vi "MSTSoftwareBinDamage.vi"() -> ()   [LabVIEW 2012]
uses:
  <vilib>/addons/database/Auxilliary.llb/DB Tools Cursor Type.ctl
  <vilib>/addons/database/Connection.llb/DB Tools Open Connec (Path).vi
  <vilib>/addons/database/Connection.llb/Conn Execute.vi
  <vilib>/addons/database/Recordset.llb/Rec Fetch Recordset Data (R).vi
  <vilib>/addons/database/Recordset.llb/Rec Destroy - Connection.vi
  <vilib>/addons/database/Recordset.llb/Rec Fetch Integer Data (R).vi
  <vilib>/addons/database/_DB Variant To Data/Database Variant To Data.xnode
  <vilib>/addons/database/NI_Database_API.lvlib
panel:
  out "concatenated string 3":string
  out "concatenated string 2":string
  out "concatenated string":string
  out "error out 2":errorcluster
  out "recordset data":variant[][](array[variant])
  out "data":string
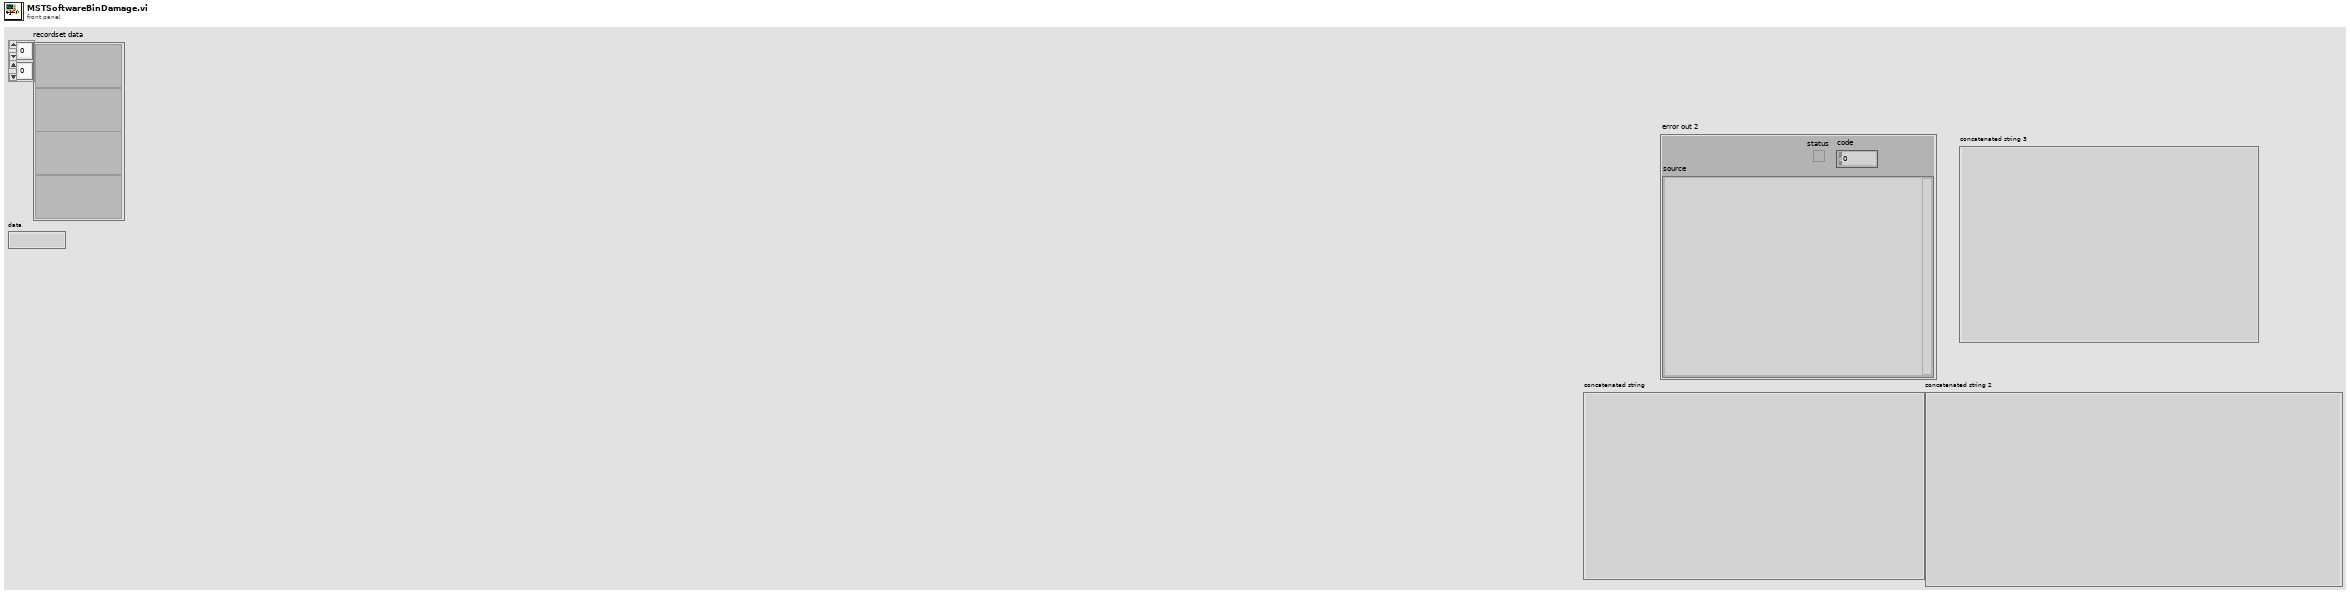
[diagram p1: front panel]
types:
  T1 = typedef "NI_Database_API.lvlib/DB Tools Cursor Type.ctl" = enum16{"forward-only", "keyset", "dynamic", "static"}
  T2 = typedef "NI_Database_API.lvlib/Conn ObjectReference.ctl" = refnum<k1>
  T3 = typedef "NI_Database_API.lvlib/Rec ObjectReference.ctl" = refnum<k1>
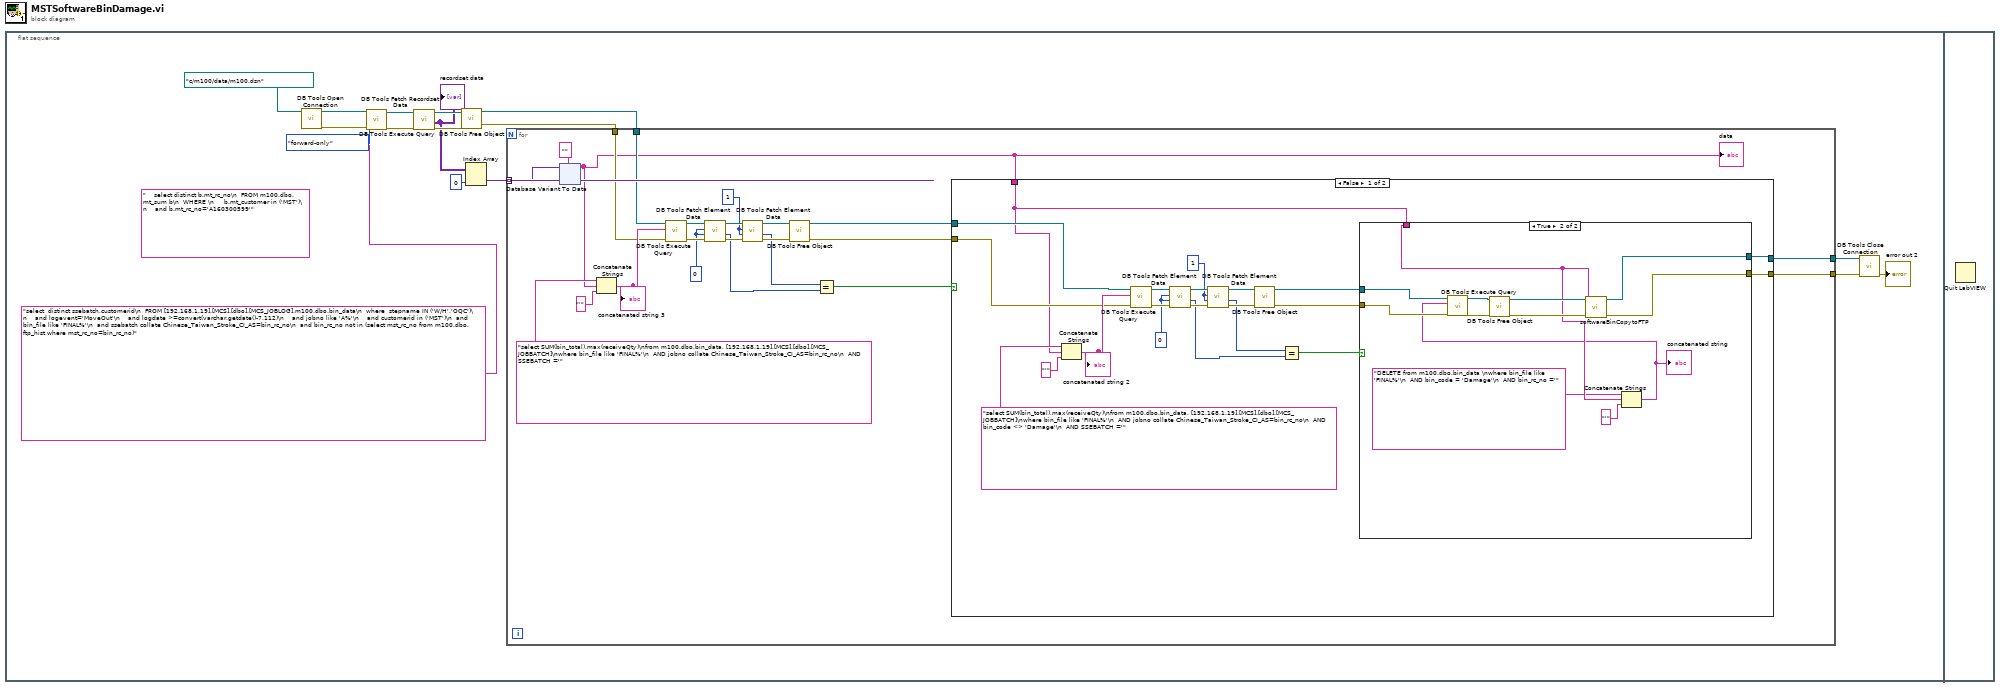
[diagram p0: block diagram]
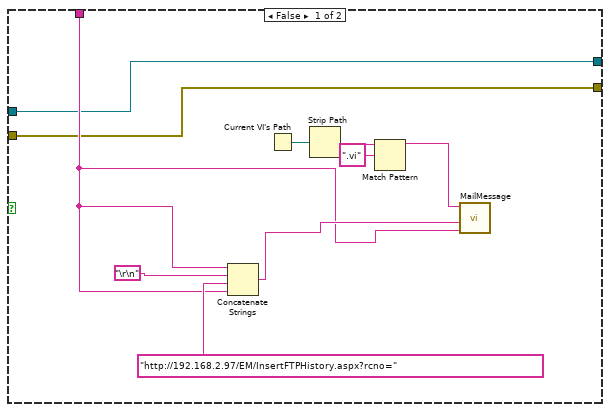
[diagram p2: hidden frame]
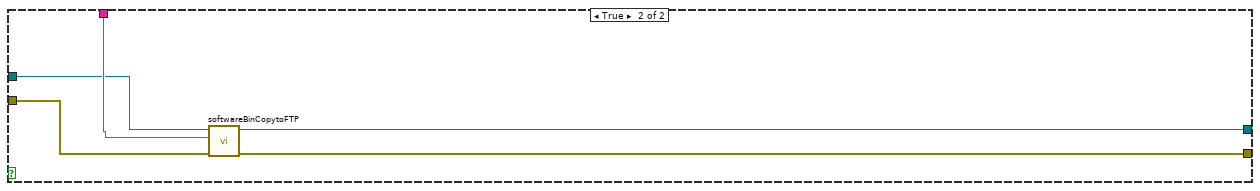
[diagram p3: hidden frame]
diagram:
  n1 = flat-sequence {
    frame #0 {
      (unwired) "    select distinct b.mt_rc_no\n  FROM m100.dbo.mt_sum b\n  WHERE \n     b.mt_customer in ('MST')\n    and b.mt_rc_no='A160300599'" ("SQL query")
      n2 = call-poly <vilib>:"DB Tools Open Connection.vi"("connection information"=path "c:/m100/data/m100.dsn") -> ("error out"=w14:errorcluster, "connection reference"=w17:T2)  [unwired: 7 in]
      n3 = call-poly <vilib>:"DB Tools Execute Query.vi"("error in (no error)"=w14, "cursor type"=DB_Tools_Cursor_Type."forward-only", "SQL query"="select  distinct ssebatch,customerid\n  FROM [192.168.1.19].[MCS].[dbo].[MCS_JOBLOG],m100.dbo.bin_data\n  where  stepname IN ('W/H','OQC')\n    and logevent='MoveOut'\n    and logdate >=convert(varchar,getdate()-7,112)\n    and jobno like 'A%'\n    and customerid in ('MST')\n  and bin_file like 'FINAL%'\n  and ssebatch collate Chinese_Taiwan_Stroke_CI_AS=bin_rc_no\n  and bin_rc_no not in (select mst_rc_no from m100.dbo.ftp_hist where mst_rc_no=bin_rc_no)", "connection reference"=w17) -> ("error out"=w13:errorcluster, "recordset reference"=w16:T3)  [unwired: 4 in]
      n4 = call-poly <vilib>:"DB Tools Fetch Recordset Data.vi"("error in (no error)"=w13, "recordset reference"=w16) -> ("error out"=w12:errorcluster, "recordset data"=w9:variant[][], "recordset reference out"=w15:T3)  [unwired: 3 in]
      "recordset data" <- w9
      n5 = call-poly <vilib>:"DB Tools Free Object.vi"("error in (no error)"=w12, "recordset reference"=w15) -> ("error out"=w5:errorcluster, "connection reference"=w6:T2)  [unwired: 8 in]
      n6 = Index Array(array=w9, index (col)=0 ("disabled index (col)")) -> (element=w7:variant[])  [unwired: 1 in]
      n7 = for {
        tunnel: w7 -> [w40] mode=indexing
        tunnel: w6 -> [w27]
        tunnel: w5 -> [w26]
        tunnel: [w19] -> w3
        tunnel: [w18] -> w2
        w31 = 1
        w32 = 0
        n8 = xnode "Database Variant To Data"("database variant"=w40, "type"="") -> ("data"=w22:string)  [unwired: 1 in, 1 out]
        "data" <- w22
        n9 = Concatenate Strings("select SUM(bin_total),max(receiveQty)\nfrom m100.dbo.bin_data, [192.168.1.19].[MCS].[dbo].[MCS_JOBBATCH]\nwhere bin_file like 'FINAL%'\n  AND jobno collate Chinese_Taiwan_Stroke_CI_AS=bin_rc_no\n  AND SSEBATCH ='" ("SQL query"), w22, "'" ("string")) -> (w28:string)
        "concatenated string 3" <- w28
        n10 = call-poly <vilib>:"DB Tools Execute Query.vi"("error in (no error)"=w26, "SQL query"=w28, "connection reference"=w27) -> ("error out"=w37:errorcluster, "recordset reference"=w38:T3)  [unwired: 5 in]
        n11 = call-poly <vilib>:"DB Tools Fetch Element Data.vi"("error in (no error)"=w37, "type"=w32, "column index"=w32, "recordset reference"=w38) -> ("error out"=w35:errorcluster, "data"=w24:i32, "recordset reference out"=w36:T3)  [unwired: 3 in]
        n12 = call-poly <vilib>:"DB Tools Fetch Element Data.vi"("error in (no error)"=w35, "type"=w31, "column index"=w31, "recordset reference"=w36) -> ("error out"=w33:errorcluster, "data"=w25:i32, "recordset reference out"=w34:T3)  [unwired: 3 in]
        n13 = call-poly <vilib>:"DB Tools Free Object.vi"("error in (no error)"=w33, "recordset reference"=w34) -> ("error out"=w20:errorcluster, "connection reference"=w21:T2)  [unwired: 8 in]
        n14 = Equal?(x=w25, y=w24) -> (x = y?=w23:bool)
        n15 = case shown="False" w23 {
          tunnel: w22 -> [w45 w88]
          tunnel: w21 -> [w48 w87]
          tunnel: w20 -> [w47 w86]
          tunnel: [w42 w85] -> w19
          tunnel: [w41 w84] -> w18
          frame False {
            w54 = 1
            w55 = 0
            n16 = Concatenate Strings("select SUM(bin_total),max(receiveQty)\nfrom m100.dbo.bin_data, [192.168.1.19].[MCS].[dbo].[MCS_JOBBATCH]\nwhere bin_file like 'FINAL%'\n  AND jobno collate Chinese_Taiwan_Stroke_CI_AS=bin_rc_no\n  AND bin_code <> 'Damage'\n  AND SSEBATCH ='" ("SQL query"), w45, "'" ("string")) -> (w51:string)
            "concatenated string 2" <- w51
            n17 = call-poly <vilib>:"DB Tools Execute Query.vi"("error in (no error)"=w47, "SQL query"=w51, "connection reference"=w48) -> ("error out"=w60:errorcluster, "recordset reference"=w61:T3)  [unwired: 5 in]
            n18 = call-poly <vilib>:"DB Tools Fetch Element Data.vi"("error in (no error)"=w60, "type"=w55, "column index"=w55, "recordset reference"=w61) -> ("error out"=w58:errorcluster, "data"=w49:i32, "recordset reference out"=w59:T3)  [unwired: 3 in]
            n19 = call-poly <vilib>:"DB Tools Fetch Element Data.vi"("error in (no error)"=w58, "type"=w54, "column index"=w54, "recordset reference"=w59) -> ("error out"=w56:errorcluster, "data"=w50:i32, "recordset reference out"=w57:T3)  [unwired: 3 in]
            n20 = call-poly <vilib>:"DB Tools Free Object.vi"("error in (no error)"=w56, "recordset reference"=w57) -> ("error out"=w43:errorcluster, "connection reference"=w44:T2)  [unwired: 8 in]
            n21 = Equal?(x=w50, y=w49) -> (x = y?=w46:bool)
            n22 = case shown="True" w46 {
              tunnel: w45 -> [w64 w74]
              tunnel: w44 -> [w63 w81]
              tunnel: w43 -> [w62 w78]
              tunnel: [w63 w83] -> w42
              tunnel: [w62 w82] -> w41
              frame False {
                n23 = Concatenate Strings(w64, "\r\n", "http://192.168.2.97/EM/InsertFTPHistory.aspx?rcno=" ("string"), w64) -> (w65:string)
                n24 = Current VI's Path() -> (path=w69:path)
                n25 = Strip Path(path=w69) -> (name=w68:string)  [unwired: 1 out]
                n26 = Match Pattern(string=w68, regular expression=".vi") -> (before substring=w66:string)  [unwired: 1 in, 3 out]
                n27 = call "MailMessage.vi"("AddSubject"=w64, "message"=w65, "program"=w66) -> ()  [unwired: 9 in]
              }
              frame True {
                n28 = Concatenate Strings("DELETE from m100.dbo.bin_data \nwhere bin_file like 'FINAL%'\n  AND bin_code = 'Damage'\n  AND bin_rc_no ='" ("SQL query"), w74, "'" ("string")) -> (w73:string)
                "concatenated string" <- w73
                n29 = call-poly <vilib>:"DB Tools Execute Query.vi"("error in (no error)"=w78, "SQL query"=w73, "connection reference"=w81) -> ("error out"=w77:errorcluster, "recordset reference"=w80:T3)  [unwired: 5 in]
                n30 = call-poly <vilib>:"DB Tools Free Object.vi"("error in (no error)"=w77, "recordset reference"=w80) -> ("error out"=w76:errorcluster, "connection reference"=w79:T2)  [unwired: 8 in]
                n31 = call "softwareBinCopytoFTP.vi"("error in (no error)"=w76, "RCNO"=w74, "connection reference 2"=w79) -> ("error out"=w82:errorcluster, "connection reference"=w83:T2)  [unwired: 7 in]
              }
            }
          }
          frame True {
            n32 = call "softwareBinCopytoFTP.vi"("error in (no error)"=w86, "RCNO"=w88, "connection reference 2"=w87) -> ("error out"=w84:errorcluster, "connection reference"=w85:T2)  [unwired: 7 in]
          }
        }
      }
      n33 = call <vilib>:"DB Tools Close Connection.vi"("error in (no error)"=w2, "connection reference"=w3) -> ("error out"=→"error out 2":errorcluster)  [unwired: 5 in]
    }
    frame #1 {
      n34 = Quit LabVIEW() -> ()  [unwired: 1 in]
    }
  }
